vi "Create Lib if not Present.vi"(7 "plug-in name":string, 8 "error in":errorcluster, 9 "dest directory":path, 10 "project ref":refnum<vi>, 11 "virtual folder ref":refnum<vi>) -> (0 "error out":errorcluster, 3 "library refnum":refnum<vi>)   [LabVIEW 2021, in "Multiple Converter.lvlib"]
uses:
  Multiple Converter.lvlib
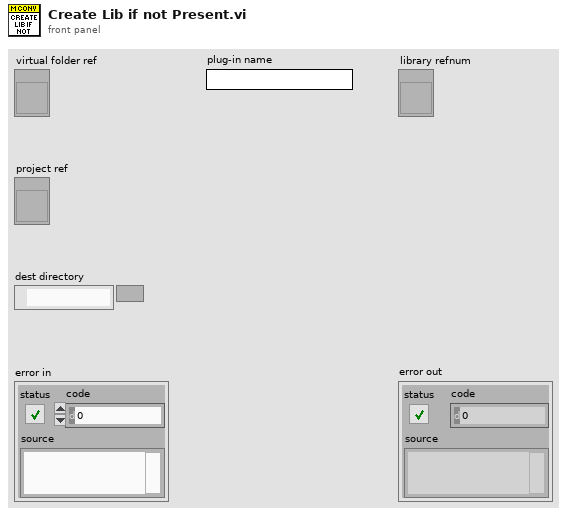
[diagram p1: front panel]
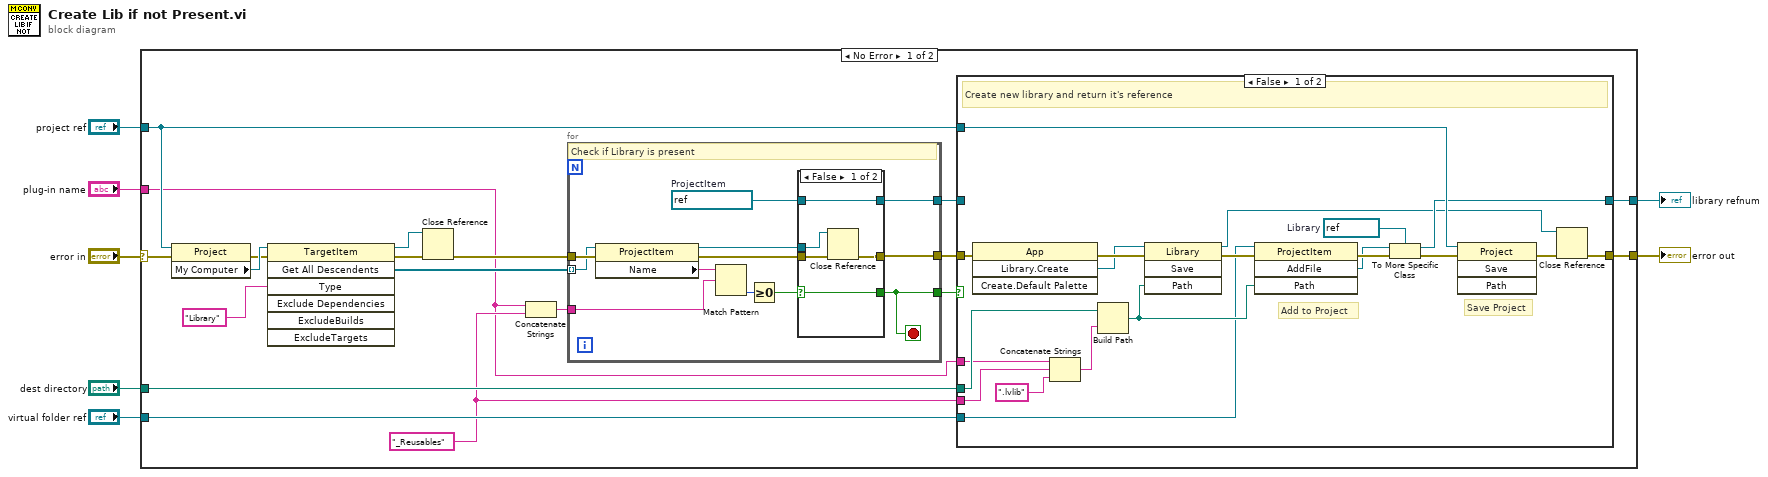
[diagram p0: block diagram]
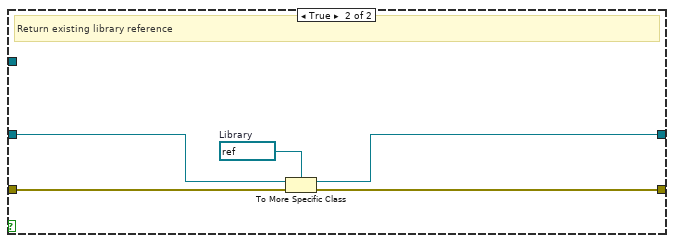
[diagram p2: hidden frame]
diagram:
  n1 = case shown="No Error" "error in" {
    selector: "error in" -> [w16 w72]
    tunnel: "dest directory" -> [w15 _]
    tunnel: "virtual folder ref" -> [w14 _]
    tunnel: "project ref" -> [w13 _]
    tunnel: [w12 w72] -> w3
    tunnel: [w10 _] -> w2
    tunnel: "plug-in name" -> [w8 _]
    frame No Error {
      w9 = "_Reusables" ("string")
      n2 = property class="Project"(reference=w13, error in=w16) -> (error out=w22:errorcluster, "My Computer"=w26:refnum<vi>)  [unwired: 1 out]
      n3 = invoke class="TargetItem" method="Get All Descendents"(reference=w26, error in=w22, "Type"="Library") -> (reference out=w23:refnum<vi>, error out=w24:errorcluster, "All Descendents"=w21:refnum<vi>[])  [unwired: 4 in, 4 out]
      n4 = Close Reference(reference=w23, error in (no error)=w24) -> (error out=w20:errorcluster)
      n5 = Concatenate Strings(w8, w9) -> (w19:string)
      n6 = for {
        tunnel: w21 -> [w62] mode=indexing
        tunnel: w20 -> [w63]
        tunnel: [w55] -> w11
        tunnel: [w54] -> w17
        tunnel: w19 -> [w53]
        tunnel: [w52] -> w18
        stop <- w52 stop-if-true
        w58 = refnum<vi> refnum  # ProjectItem
        # "Check if Library is present"
        n7 = property class="ProjectItem"(reference=w62, error in=w63) -> (reference out=w57:refnum<vi>, error out=w56:errorcluster, "Name"=w61:string)
        n8 = Match Pattern(string=w61, regular expression=w53) -> (offset past match=w60:i32)  [unwired: 1 in, 3 out]
        n9 = Greater Or Equal To 0?(x=w60) -> (x >= 0?=w59:bool)
        n10 = case shown="False" w59 {
          selector: w59 -> [w65 w70]
          tunnel: w57 -> [w66 w71]
          tunnel: [w68 w69] -> w54
          tunnel: [w67 w71] -> w55
          tunnel: w58 -> [w67 _]
          tunnel: [w65 w70] -> w52
          tunnel: w56 -> [w64 w69]
          frame False {
            n11 = Close Reference(reference=w66, error in (no error)=w64) -> (error out=w68:errorcluster)
          }
          frame True {
          }
        }
      }
      n12 = case shown="False" w18 {
        tunnel: w17 -> [w46 w51]
        tunnel: w15 -> [w44 _]
        tunnel: w14 -> [w38 _]
        tunnel: w13 -> [w37 _]
        tunnel: [w31 w50] -> w12
        tunnel: w11 -> [_ w48]
        tunnel: [w32 w49] -> w10
        tunnel: w9 -> [w28 _]
        tunnel: w8 -> [w27 _]
        frame False {
          w33 = refnum<vi> refnum  # Library
          # "Save Project"
          # "Add to Project"
          # "Create new library and return it's reference"
          n13 = invoke class="App" method="Library.Create"(error in=w46) -> (error out=w45:errorcluster, "Create Library"=w42:refnum<vi>)  [unwired: 3 in, 2 out]
          n14 = Concatenate Strings(w27, w28, ".lvlib" ("string")) -> (w43:string)
          n15 = Build Path(base path=w44, name or relative path=w43) -> (appended path=w39:path)
          n16 = invoke class="Library" method="Save"(reference=w42, error in=w45, "Path"=w39) -> (reference out=w30:refnum<vi>, error out=w40:errorcluster)  [unwired: 1 in, 2 out]
          n17 = invoke class="ProjectItem" method="AddFile"(reference=w38, error in=w40, "Path"=w39) -> (error out=w41:errorcluster, "AddFile"=w34:refnum<vi>)  [unwired: 1 in, 2 out]
          n18 = To More Specific Class(target class=w33, reference=w34, error in=w41) -> (specific class reference=w32:refnum<vi>, error out=w35:errorcluster)
          n19 = invoke class="Project" method="Save"(reference=w37, error in=w35) -> (error out=w36:errorcluster)  [unwired: 2 in, 3 out]
          n20 = Close Reference(reference=w30, error in (no error)=w36) -> (error out=w31:errorcluster)
        }
        frame True {
          w47 = refnum<vi> refnum  # Library
          # "Return existing library reference"
          n21 = To More Specific Class(target class=w47, reference=w48, error in=w51) -> (specific class reference=w49:refnum<vi>, error out=w50:errorcluster)
        }
      }
    }
    frame Error {
    }
  }
  "error out" <- w3
  "library refnum" <- w2
